vi "Sub_FGV_Serial.vi"(6 "Read Count":u32=1000, 7 "상태":T2, 8 "Error In":errorcluster caption="에러 입력", 9 "Command":string="*IDN?", 10 "Serial Settings":T1={"baud rate"=9600, "data bits"=8, "parity"=enum."None", "stop bits"=10, "flow control"=0} {"flow control" items=["None"=0, "XON/XOFF"=1, "RTS/CTS"=2, "DTR/DSR"=4]; "stop bits" items=["1.0"=10, "1.5"=15, "2.0"=20]; "data bits" min=5 max=8 step=1; "baud rate" items=["75"=75, "110"=110, "134"=134, "150"=150, "300"=300, "600"=600, "1200"=1200, "1800"=1800, "2400"=2400, "4800"=4800, "7200"=7200, "9600"=9600, "14400"=14400, "19200"=19200, "28800"=28800, "38400"=38400, "56000"=56000, "57600"=57600, "115200"=115200, "128000"=128000, "230400"=230400]}, 11 "VISA resource name":refnum<visa-resource-name>="COM1") -> (0 "Error Out":errorcluster caption="에러 출력", 2 "Response":string)   [LabVIEW 2019]
uses:
  Program Files (x86)/National Instruments/LabVIEW 2019/examples/Instrument IO/Serial/support/Serial - Settings.ctl
  <vilib>/Instr/_visa.llb/VISA Configure Serial Port (Instr).vi
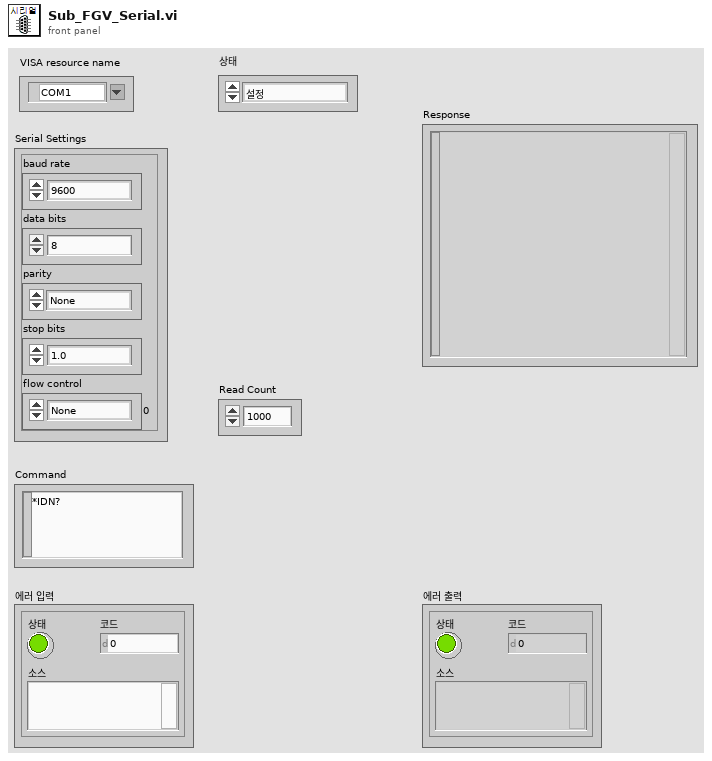
[diagram p1: front panel]
types:
  T1 = typedef "Serial - Settings.ctl" = cluster{"baud rate":u32, "data bits":u16, "parity":enum16{"None", "Odd", "Even", "Mark", "Space"}, "stop bits":u16, "flow control":u16}
  T2 = typedef "상태.ctl" = enum16{"설정", "읽기", "쓰기", "닫기"}
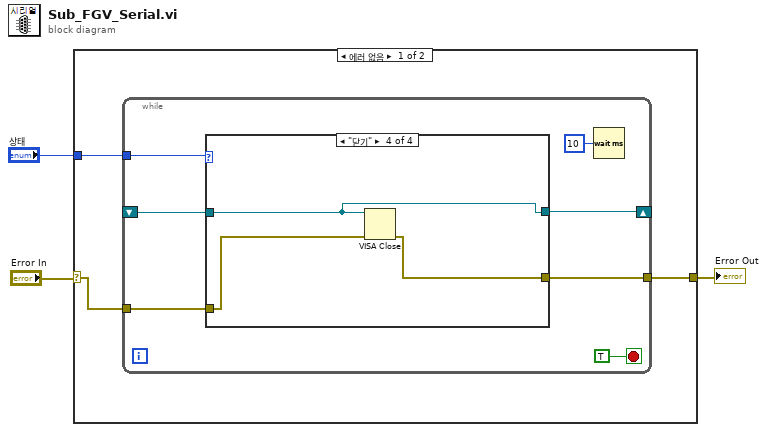
[diagram p0: block diagram]
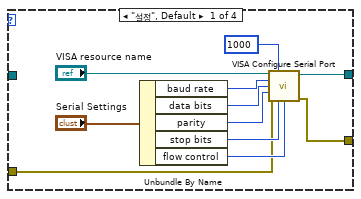
[diagram p2: hidden frame]
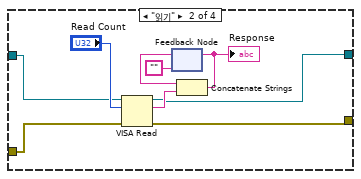
[diagram p3: hidden frame]
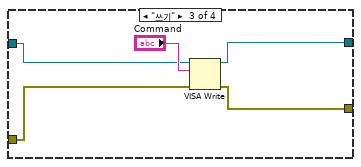
[diagram p4: hidden frame]
diagram:
  n1 = case shown="에러 없음" "Error In" {
    selector: "Error In" -> [w5 w42]
    tunnel: "상태" -> [w6 _]
    tunnel: [w4 w42] -> w1
    frame No Error {
      n2 = while {
        shift-right: [w10] -> _
        shift-left: _ -> [w9]
        tunnel: w6 -> [w13]
        tunnel: w5 -> [w8]
        tunnel: [w7] -> w4
        stop <- TRUE stop-if-true
        n3 = case shown="\"닫기\"" w13 {
          tunnel: [w16 w27 w36 w41] -> w10
          tunnel: w9 -> [_ w28 w37 w41]
          tunnel: w8 -> [w15 w26 w35 w40]
          tunnel: [w14 w25 w34 w39] -> w7
          frame "설정", Default {
            n4 = Unbundle By Name("Serial Settings") -> ("baud rate"=w19:u32, "data bits"=w23:u16, "parity"=w22:enum16{"None", "Odd", "Even", "Mark", "Space"}, "stop bits"=w20:u16, "flow control"=w21:u16)
            n5 = call-poly "VISA Configure Serial Port"("VISA resource name"="VISA resource name", "timeout (10sec)"=u32 1000, "baud rate (9600)"=w19, "data bits (8)"=w23, "parity (0:none)"=w22, "error in (no error)"=w15, "stop bits (10: 1 bit)"=w20, "flow control (0:none)"=w21) -> ("VISA resource name out"=w16:refnum<visa-resource-name>, "error out"=w14:errorcluster)  [unwired: 6 in]
          }
          frame "읽기" {
            n6 = VISA Read(VISA resource name=w28, byte count="Read Count", error in (no error)=w26) -> (VISA resource name out=w27:refnum<visa-resource-name>, read buffer=w32:string, error out=w25:errorcluster)  [unwired: 1 out]
            n7 = feedback #1("") -> (w31:string)
            n8 = Concatenate Strings(w31, w32) -> (w30:string)
            "Response" <- w30
            n9 = feedback-in #1(w30) -> ()
          }
          frame "쓰기" {
            n10 = VISA Write(VISA resource name=w37, write buffer="Command", error in (no error)=w35) -> (VISA resource name out=w36:refnum<visa-resource-name>, error out=w34:errorcluster)  [unwired: 1 out]
          }
          frame "닫기" {
            n11 = VISA Close(VISA resource name=w41, error in (no error)=w40) -> (error out=w39:errorcluster)
          }
        }
        n12 = Wait (ms)(milliseconds to wait=u32 10 ("대기 시간 (ms)")) -> ()  [unwired: 1 out]
      }
    }
    frame Error {
    }
  }
  "Error Out" <- w1
